vi "Robot Global Data.vi"() -> ()   [LabVIEW 2017]
doc: "This global VI can contain as many global variables as you need. Place a control on the panel, give it a good name. To read or write to it from a VI, drag the icon to the diagram of that VI. You can also drag from the project. Click on the node to change which global you access. You shouldn't have multiple locations writing to a global or it will cause a race-condition."
uses:
  <vilib>/Rock Robotics/WPI/Camera/WPI_CameraImageSize.ctl
  <vilib>/Rock Robotics/WPI/DriverStation/WPI_DriverStationRobotMode2.ctl
panel:
  in  "Pivot":enum16{"High", "Mid", "Low"}(ring)
  in  "Pivot Power":dbl
  in  "Track":bool
  in  "Y Velocity":dbl
  in  "X Velocity":dbl
  in  "Reset Encoders":bool
  in  "Y Distance":dbl
  in  "X Distance":dbl
  in  "Turret Power":dbl
  in  "ArmExtend":dbl
  in  "Lift":enum16{"Low", "Switch", "Mid", "High"}(ring)
  in  "Offset":bool
  in  "Reset Gyro":bool
  in  "Robot Centric":bool
  in  "z":dbl
  in  "y":dbl
  in  "x":dbl
  in  "Robot Mode":T1
  in  "image size":T2=enum."320x240"
  in  "Enable Vision":bool
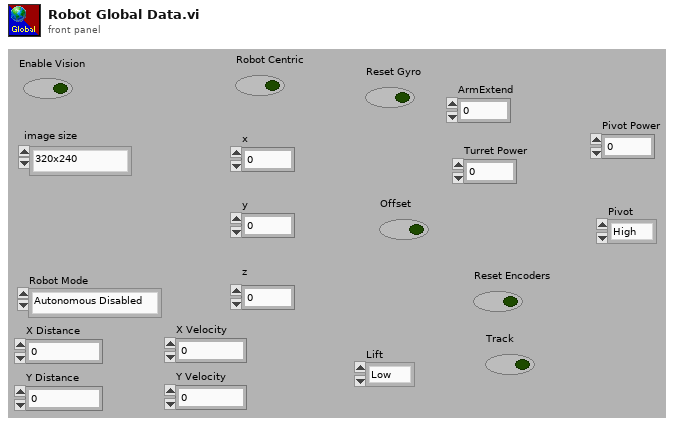
[diagram p1: front panel]
types:
  T1 = typedef "WPI_DriverStationRobotMode2.ctl" = enum16{"Autonomous Disabled", "Autonomous Enabled", "Teleop Disabled", "Teleop Enabled", "Disconnected", "Finish", "Test Disabled", "Test Enabled", "Emergency Stopped"}
  T2 = typedef "WPI_CameraImageSize.ctl" = enum16{"640x480", "320x240", "160x120", "Custom"}
diagram:
